vi "Test Get Lifecycle Started.vi"(8 "error in (no error)":errorcluster, 11 "Debug State Analyzer Test In":refnum<class "Debug State Analyzer Test.lvclass">) -> (0 "error out":errorcluster, 3 "Debug State Analyzer Test Out":refnum<class "Debug State Analyzer Test.lvclass">)   [LabVIEW 2020, in "Debug State Analyzer Test.lvclass"]
uses:
  Debug State Analyzer Test.lvclass
  C:/Program Files (x86)/National Instruments/LabVIEW 2020/vi.lib/Astemes/LUnit/Test Case.lvclass
  source/Debug Data/Raw Debug Data.ctl
  source/State Analyzer/Debug State Analyzer.lvclass
  <vilib>/Astemes/LUnit/Test Case.lvclass/Test Case.ctl
  <vilib>/Astemes/LUnit/LUnit Assertion Result.lvclass/LUnit Assertion Result.ctl
  <vilib>/Astemes/LUnit/LUnit Test Case Result.lvclass/LUnit Test Case Result.ctl
  <vilib>/Astemes/LUnit/LUnit Method Result.lvclass/LUnit Method Result.ctl
  01074fa8-ee8a-411d-bc8b-fc92c4f90959.vi
  <vilib>/Astemes/LUnit/Palette/Pass.vi
  <vilib>/Astemes/LUnit/Palette/Fail.vi
  <vilib>/Astemes/LUnit/Compare Variants.vi
  <vilib>/Astemes/LUnit/Describe Comparison.vi
  <vilib>/Astemes/LUnit/Set Assertion Type.vi
  <vilib>/Astemes/LUnit/Add test result.vi
  <vilib>/Astemes/LUnit/LUnit Write Passed.vi
  <vilib>/Astemes/LUnit/LUnit Write Message.vi
  <vilib>/Astemes/LUnit/LUnit Write Description.vi
  <vilib>/Astemes/LUnit/Variant to string.vi
  <vilib>/Astemes/LUnit/LUnit Write Assertion Type.vi
  <vilib>/Astemes/LUnit/LUnit Record Assertion Result.vi
  <vilib>/Astemes/LUnit/LUnit Aggregate Assertion Results.vi
  <vilib>/Astemes/LUnit/Assertion Result/LUnit Read Status.vi
  <vilib>/Astemes/LUnit/LUnit Read Message.vi
  <vilib>/Astemes/LUnit/LUnit Read Description.vi
  <vilib>/Astemes/LUnit/Method Result/LUnit Merge Status.vi
  <vilib>/Astemes/LUnit/LUnit Concatenate result strings.vi
  <vilib>/Utility/Data Type/Get Type Information.vi
  <vilib>/Utility/LVClass/Get LV Class Name.vi
  <vilib>/Astemes/LUnit/LUnit Assertion Result.lvclass
  Debug State Analyzer Test.lvclass/Debug State Analyzer Test.ctl
  source/Debug Data/Debug Data.lvclass
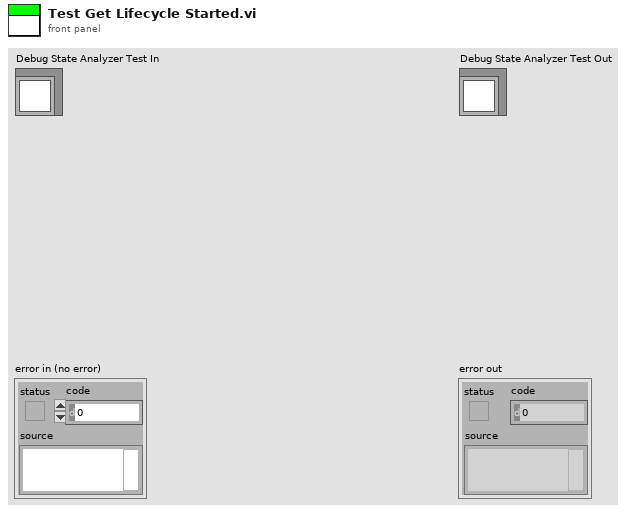
[diagram p1: front panel]
types:
  T1 = typedef "Debug Data.lvclass/Raw Debug Data.ctl" = cluster{"Action":string, "Call Chain":string, "Process":string, "Message":string, "Message Data":variant, "Time":dbl}
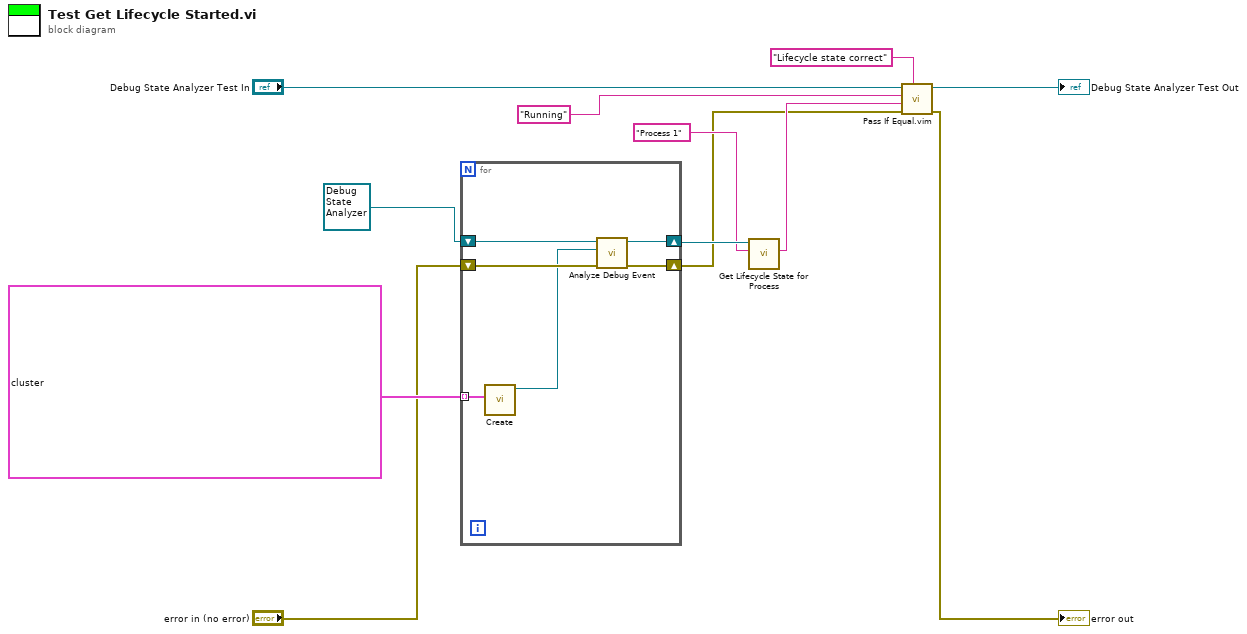
[diagram p0: block diagram]
diagram:
  n1 = for {
    tunnel: T1[] [{"Action"="Send", "Call Chain"="Test.vi:123456", "Process"="Process 1", "Message"="Init", "Message Data"=variant, "Time"=0.0}, {"Action"="Receive", "Call Chain"="TF.lvlib:Process.lvclass:Handle Messages.vi:1960001", "Process"="Process 1", "Message"="Init", "Message Data"=variant, "Time"=0.0}, {"Action"="Send", "Call Chain"="Test.vi", "Process"="Process 1", "Message"="Start", "Message Data"=variant, "Time"=0.0}, {"Action"="Receive", "Call Chain"="Test.vi", "Process"="Process 1", "Message"="Start", "Message Data"=variant, "Time"=0.0}] ("Debug Data Cluster") -> [w18] mode=indexing
    shift-right: [w16] -> w5
    shift-left: refnum<class "Debug State Analyzer.lvclass"> refnum ("Debug State Analyzer in") -> [w17]
    shift-right: [w14] -> w2
    shift-left: "error in (no error)" -> [w15]
    n2 = call "Create.vi"("Debug Data Cluster"=w18) -> ("Debug Data out"=w13:refnum<class "Debug Data.lvclass">)  [unwired: 9 in, 1 out]
    n3 = call "Analyze Debug Event.vi"("error in (no error)"=w15, "Debug Data.lvclass"=w13, "Debug State Analyzer In"=w17) -> ("error out"=w14:errorcluster, "Debug State Analyzer Out"=w16:refnum<class "Debug State Analyzer.lvclass">)  [unwired: 7 in]
  }
  n4 = call "Get Lifecycle State for Process.vi"("Process"="Process 1", "Debug State Analyzer In"=w5) -> ("Lifecycle State"=w3:string)  [unwired: 8 in, 1 out]
  n5 = call "Pass If Equal.vim"("Description"="Lifecycle state correct", "error in (no error)"=w2, "Actual"=w3, "Expected"="Running", "LUnit Test Case In"="Debug State Analyzer Test In") -> ("error out"=→"error out":errorcluster, "LUnit Test Case Out"=→"Debug State Analyzer Test Out":refnum<class "Debug State Analyzer Test.lvclass">)  [unwired: 5 in]
